vi "RPC Method MeasurementService Measure Logic.vi"(8 "error in":errorcluster, 11 "gRPCid in":T1) -> (0 "error out":errorcluster)   [LabVIEW 2020, in "LoadRegulation.lvlib" / "MeasurementService.lvclass"]
uses:
  MeasurementService.lvclass
  MeasurementService.lvclass/MeasurementService.ctl
  6e93e594-9b53-4a41-bad0-565312cbf1e4.vi
  <vilib>/gRPC/LabVIEW gRPC Library/grpc-lvsupport-release.lvlib
  <vilib>/gRPC/LabVIEW gRPC Library/Server API/typeDefs/gRPC Status Code.ctl
  c01dd925-8d21-4ce6-b452-e7218c44af5c.vi
  LoadRegulation.lvlib
  Measurement Configuration.ctl
  MeasurementContext/MeasurementContext.lvclass
  <vilib>/gRPC/LabVIEW gRPC Library/Shared/grpcId.ctl
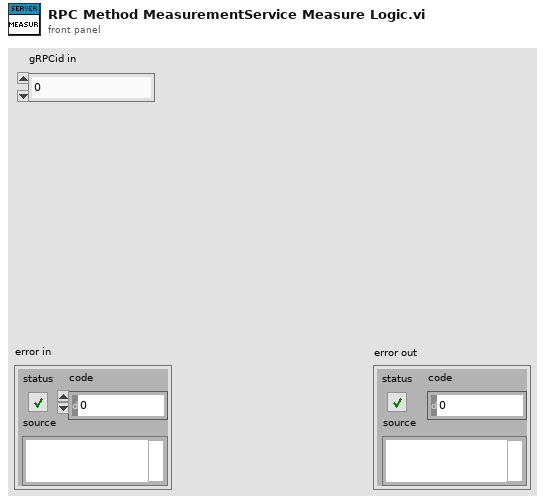
[diagram p1: front panel]
types:
  T1 = typedef "grpc-lvsupport-release.lvlib/grpcId.ctl" = u64
  T2 = typedef "LoadRegulation.lvlib/Measurement Configuration.ctl" = cluster{"Input Voltage in V":dbl, "Nominal Output Voltage in V":dbl, "Start":dbl, "Stop":dbl, "Step":dbl, "Input SMU":string, "Load SMU":string, "Input DMM":string, "Load DMM":string}
  T3 = typedef "LoadRegulation.lvlib/ni_measurementlink_measurement_v1_MeasureRequest.ctl" = cluster{"configuration_parameters":T4, "pin_map_context":T5}
  T4 = typedef "LoadRegulation.lvlib/google_protobuf_Any.ctl" = cluster{"type_url":string, "value":u8[]}
  T5 = typedef "LoadRegulation.lvlib/ni_measurementlink_PinMapContext.ctl" = cluster{"pin_map_id":string, "sites":i32[]}
  T6 = typedef "LoadRegulation.lvlib/Measurement Results.ctl" = cluster{"Load Regulation (%)":dbl, "Load Regulation (mV/mA)":dbl, "Test Results.Load Current in A":dbl[], "Output Voltage in V":dbl[]}
  T7 = typedef "grpc-lvsupport-release.lvlib/gRPC Status Code.ctl" = enum16{"OK", "CANCELLED", "UNKNOWN", "INVALID_ARGUMENT", "DEADLINE_EXCEEDED", "NOT_FOUND", "ALREADY_EXISTS", "PERMISSION_DENIED", "RESOURCE_EXHAUSTED", "FAILED_PRECONDITION", "ABORTED", "OUT_OF_RANGE", "UNIMPLEMENTED", "INTERNAL", "UNAVAILABLE", "DATA_LOSS", "UNAUTHENTICATED"}
  T8 = typedef "grpc-lvsupport-release.lvlib/Any.ctl" = cluster{"Type Url":string, "Bytes":u8[]}
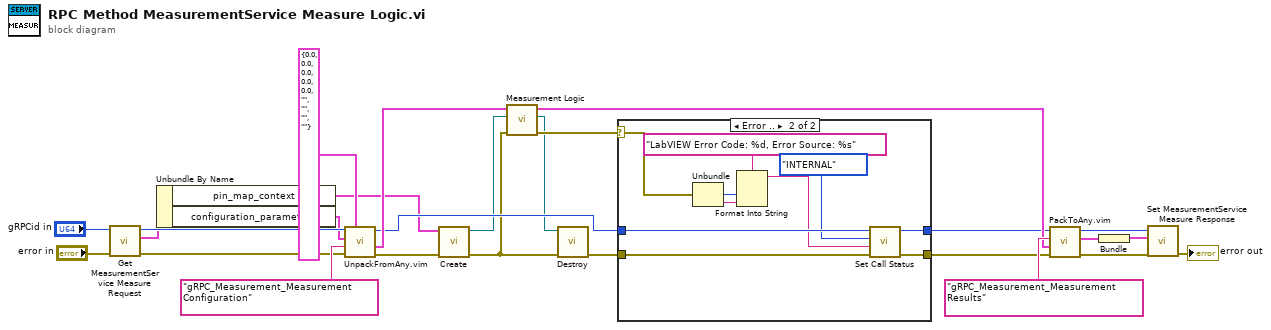
[diagram p0: block diagram]
diagram:
  n1 = call "Get MeasurementService Measure Request.vi"("error in (no error)"="error in", "gRPCid in"="gRPCid in") -> ("error out"=w8:errorcluster, "Message Data"=w9:T3, "gRPCid out"=w10:T1)  [unwired: 7 in]
  n2 = Unbundle By Name(w9) -> ("pin_map_context"=w4:T5, "configuration_parameters"=w5:T4)
  n3 = call "UnpackFromAny.vim"("Data Type"=T2 {"Input Voltage in V"=0.0, "Nominal Output Voltage in V"=0.0, "Start"=0.0, "Stop"=0.0, "Step"=0.0, "Input SMU"="", "Load SMU"="", "Input DMM"="", "Load DMM"=""} ("Measurement Configuration"), "error in"=w8, "Message Type"="gRPC_Measurement_Measurement Configuration", "Any"=w5, "gRPCid in"=w10) -> ("error out"=w6:errorcluster, "Unpacked Value"=w23:T2, "gRPCid out"=w16:u64)  [unwired: 4 in]
  n4 = call "Create.vi"("error in (no error)"=w6, "pin map context"=w4) -> ("error out"=w3:errorcluster, "MeasurementContext out"=w7:refnum<class "MeasurementContext.lvclass">)  [unwired: 8 in]
  n5 = call "Measurement Logic.vi"("error in"=w3, "Measurement Context"=w7, "Measurement Configuration"=w23) -> ("error out"=w17:errorcluster, "Measurement Context out"=w2:refnum<class "MeasurementContext.lvclass">, "Measurement Results"=w24:T6)  [unwired: 6 in]
  n6 = call-dynamic "Destroy.vi"("error in (no error)"=w3, "MeasurementContext in"=w2) -> ("error out"=w1:errorcluster)  [unwired: 9 in]
  n7 = case shown="Error .." w17 {
    selector: w17 -> [_ w38]
    tunnel: w16 -> [w28 w37]
    tunnel: [w28 w36] -> w15
    tunnel: w1 -> [w27 w34]
    tunnel: [w27 w35] -> w14
    frame No Error {
    }
    frame Error {
      n8 = Unbundle(w38) -> ("code"=w32:i32, "source"=w31:string)  [unwired: 1 out]
      n9 = Format Into String(format string="LabVIEW Error Code: %d, Error Source: %s", w32, w31) -> (resulting string=w29:string)  [unwired: 2 in, 1 out]
      n10 = call <vilib>:"Set Call Status.vi"("error in"=w34, "Details"=w29, "Status Code"=gRPC_Status_Code."INTERNAL", "gRPCid in"=w37) -> ("error out"=w35:errorcluster, "gRPCid out"=w36:T1)  [unwired: 6 in]
    }
  }
  n11 = call "PackToAny.vim"("error in"=w14, "Data To Pack"=w24, "Message Type"="gRPC_Measurement_Measurement Results", "gRPCid in"=w15) -> ("error out"=w18:errorcluster, "Any"=w20:T8, "gRPCid out"=w21:u64)  [unwired: 5 in]
  n12 = Bundle("Any"=w20) -> (w19:cluster{"Any":T8})  [unwired: 1 in]
  n13 = call "Set MeasurementService Measure Response.vi"("error in (no error)"=w18, "Message Data"=w19, "gRPCid in"=w21) -> ("error out"=→"error out":errorcluster)  [unwired: 8 in]
